vi "Read (Multiple Waveforms).vi"(8 "error in (no error)":errorcluster, 9 "Timeout (10000 ms)":u32=10000, 10 "Channels":u16[](array[ring])=[0, 1] items=["Channel 1", "Channel 2", "Channel 3", "Channel 4"], 11 "VISA resource name":refnum<visa-resource-name>) -> (0 "error out":errorcluster, 2 "Waveform Data":waveform(dbl)[](graph), 3 "VISA resource name out":refnum<visa-resource-name>)   [LabVIEW 2017, in "RIGOL DS1000 Series.lvlib"]
doc: "Initiates an acquisition on all channels that you enabled with the Configure Channel VI. The VI waits for the acquisition to complete and returns the waveform for the <B>Source Channel</B> you specified. If the oscilloscope did not complete the acquisition within the time period you specify with the <B>Timeout</B> control, the VI returns a timeout error. A common cause for a timeout error is the acquisition was not triggered. For example, the trigger level is out of range of the waveform."
uses:
  RIGOL DS1000 Series.lvlib
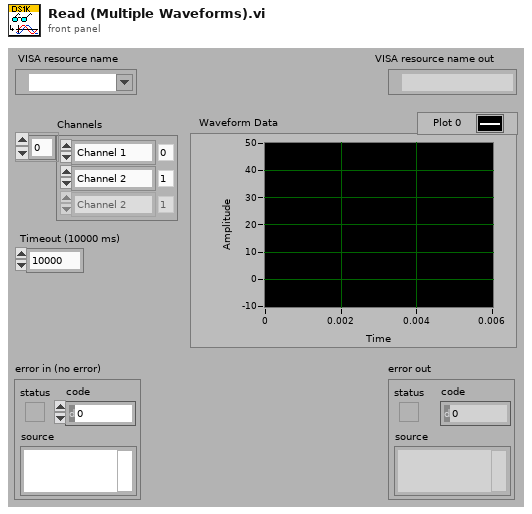
[diagram p1: front panel]
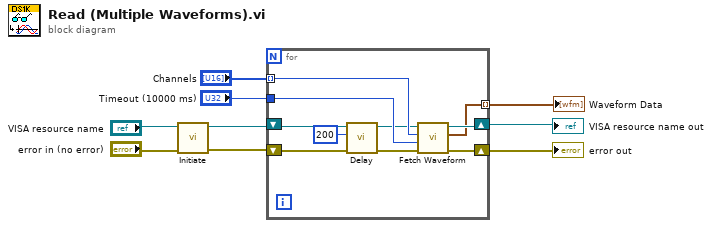
[diagram p0: block diagram]
diagram:
  n1 = call "Initiate.vi"("error in (no error)"="error in (no error)", "VISA resource name"="VISA resource name") -> ("error out"=w4:errorcluster, "VISA resource name out"=w5:refnum<visa-resource-name>)  [unwired: 8 out]
  n2 = for {
    shift-right: [w18] -> w2
    shift-left: w4 -> [w13]
    tunnel: "Channels" -> [w17] mode=indexing
    tunnel: [w16] -> w6 mode=indexing
    tunnel: "Timeout (10000 ms)" -> [w15]
    shift-right: [w19] -> w1
    shift-left: w5 -> [w14]
    n3 = call "Delay.vi"("error in (no error)"=w13, "Delay (ms)"=u32 200, "VISA resource name"=w14) -> ("error out"=w11:errorcluster, "VISA resource name out"=w12:refnum<visa-resource-name>)  [unwired: 7 out]
    n4 = call "Fetch Waveform.vi"("error in (no error)"=w11, "Timeout (10000 ms)"=w15, "Channel (0: Channel 1)"=w17, "VISA resource name"=w12) -> ("error out"=w18:errorcluster, "Waveform Data"=w16:waveform(dbl), "VISA resource name out"=w19:refnum<visa-resource-name>)  [unwired: 5 out]
  }
  "error out" <- w2
  "VISA resource name out" <- w1
  "Waveform Data" <- w6
